vi "logBtn.vi"() -> ()   [LabVIEW 2020]
uses:
  <vilib>/Utility/sysdir.llb/System Directory Type.ctl
panel:
  in  "stop":bool
  in  "C":bool
  in  "B":bool
  in  "A":bool
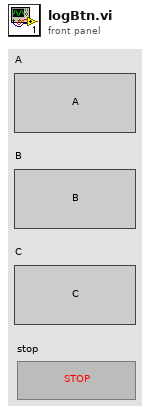
[diagram p1: front panel]
types:
  T1 = enum16{"open", "replace", "create", "open or create", "replace or create", "replace or create with confirmation"}
  T2 = typedef "System Directory Type.ctl" = i32
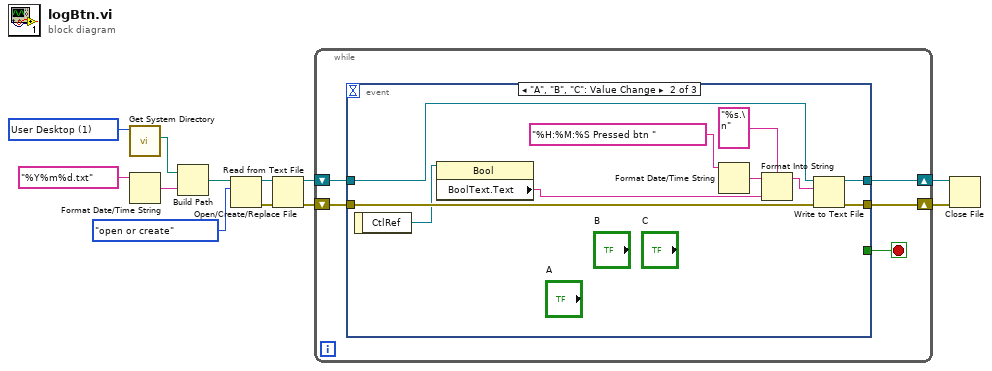
[diagram p0: block diagram]
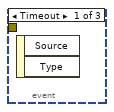
[diagram p2: hidden frame]
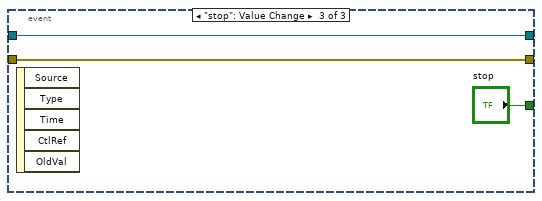
[diagram p3: hidden frame]
diagram:
  w12 = T2 1 items=["User Home"=0, "User Desktop"=1, "User Documents"=2, "User Application Data"=3, "User Preferences"=4, "User Temporary"=5, "Public Documents"=6, "Public Application Data"=7, "Public Preferences"=8, "Public Cache"=13, "System Core Libraries"=9, "System Installed Libraries"=10, "Application Files"=11, "Boot Volume Root"=12] ("system directory type")
  n1 = call <vilib>:"Get System Directory.vi"("system directory type"=w12) -> ("system directory"=w11:path)  [unwired: 10 in]
  n2 = Format Date/Time String(time format string (%c)="%Y%m%d.txt") -> (date/time string=w10:string)  [unwired: 2 in]
  n3 = Build Path(base path=w11, name or relative path=w10) -> (appended path=w8:path)
  n4 = Open/Create/Replace File(file path (use dialog)=w8, operation (0:open)=T1."open or create") -> (refnum out=w4:refnum<file>, error out=w3:errorcluster)  [unwired: 4 in, 1 out]
  n5 = Read from Text File(file (use dialog)=w4, error in=w3) -> (refnum out=w1:refnum<file>, error out=w2:errorcluster)  [unwired: 2 in, 2 out]
  n6 = while {
    shift-right: [w15] -> w6
    shift-left: w1 -> [w17]
    shift-right: [w14] -> w5
    shift-left: w2 -> [w16]
    stop <- w13 stop-if-true
    n7 = event shown="[1] \"A\", \"B\", \"C\": Value Change" {
      selector: _ -> [_ _ _]
      dyn-events: _ -> [_ _ _]
      timeout: _ -> [_ _ _]
      tunnel: w17 -> [_ w26 w29]
      tunnel: w16 -> [_ w25 w28]
      tunnel: [_ w24 w29] -> w15
      tunnel: [_ w23 w28] -> w14
      tunnel: [_ _ "stop"] -> w13
      event Timeout {
        n8 = event-data() -> ()  [unwired: 1 in, 2 out]
      }
      event "A", "B", "C": Value Change {
        n9 = event-data() -> ("CtlRef"=w20:refnum<vi>)  [unwired: 1 in]
        n10 = property class="Bool"(reference=w20) -> ("BoolText.Text"=w19:string)  [unwired: 1 in, 2 out]
        n11 = Format Date/Time String(time format string (%c)="%H:%M:%S Pressed btn ") -> (date/time string=w22:string)  [unwired: 2 in]
        n12 = Format Into String(format string="%s.\n", initial string=w22, w19) -> (resulting string=w18:string)  [unwired: 1 in, 1 out]
        n13 = Write to Text File(file (use dialog)=w26, text=w18, error in=w25) -> (refnum out=w24:refnum<file>, error out=w23:errorcluster)  [unwired: 1 in, 1 out]
      }
      event "stop": Value Change {
        n14 = event-data() -> ()  [unwired: 1 in, 5 out]
      }
    }
  }
  n15 = Close File(refnum=w6, error in=w5) -> ()  [unwired: 2 out]
